vi "pid.vi"(0 "目标":dbl, 1 "当前":dbl, 2 "kp":dbl, 3 "ki":dbl, 4 "kd":dbl) -> (5 "out":dbl)   [LabVIEW 2022 SP3]
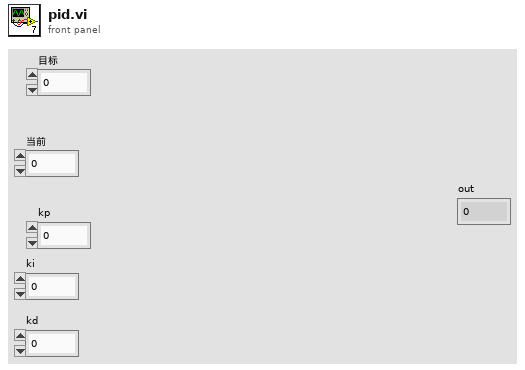
[diagram p1: front panel]
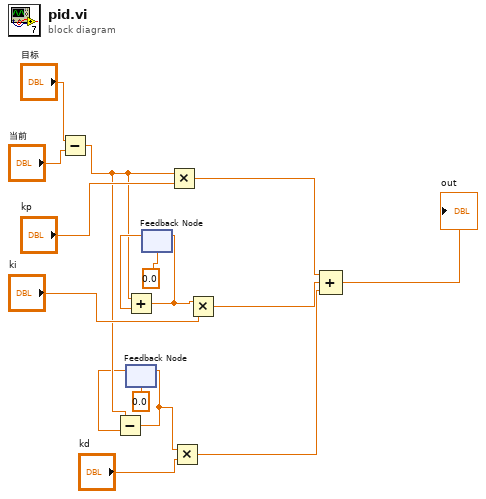
[diagram p0: block diagram]
diagram:
  n1 = Subtract(x="目标", y="当前") -> (x-y=w9:dbl)
  n2 = feedback #1(0.0) -> (w8:dbl)
  n3 = Subtract(x=w9, y=w8) -> (x-y=w6:dbl)
  n4 = feedback-in #1(w6) -> ()
  n5 = feedback #2(0.0) -> (w13:dbl)
  n6 = Add(x=w9, y=w13) -> (x+y=w11:dbl)
  n7 = feedback-in #2(w11) -> ()
  n8 = Multiply(x=w9, y="kp") -> (x*y=w4:dbl)
  n9 = Multiply(x=w6, y="kd") -> (x*y=w2:dbl)
  n10 = Multiply(x=w11, y="ki") -> (x*y=w3:dbl)
  n11 = Compound Arithmetic op=ADD(w4, w3, w2) -> (→"out":dbl)
